vi "DegToDAC (SubVI).vi"(8 "error in (no error)":errorcluster, 10 "R2":dbl format="%#_13g", 11 "Numeric":dbl) -> (0 "error out":errorcluster, 2 "output array":u8[](array[numeric]))   [LabVIEW 2017]
uses:
  <vilib>/express/express arith-compare/Formula/XNode/ExpressFormulaBlockNode.xnode
panel:
  in  "Array":dbl[](array[numeric])=[1202.0, 1288.0, 1472.0, 1472.0, 1379.0]
  out "Result":dbl
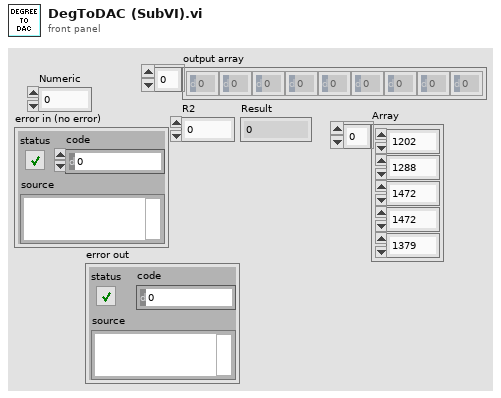
[diagram p1: front panel]
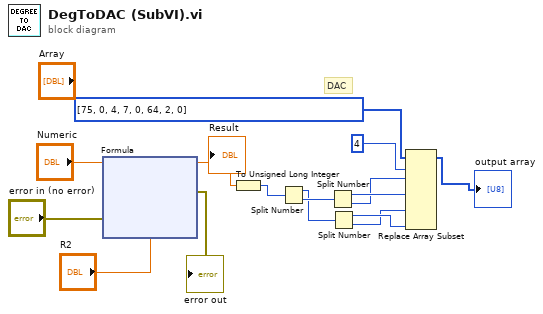
[diagram p0: block diagram]
diagram:
  # "DAC"
  n1 = xnode "Formula"("X2"="R2", "X1"="Numeric", "error in (no error)"="error in (no error)") -> ("Result"=w2:dbl, "error out"=→"error out":errorcluster)
  "Result" <- w2
  n2 = To Unsigned Long Integer(number=w2) -> (unsigned 32bit integer=w3:u32)
  n3 = Split Number(x=w3) -> (hi(x)=w9:u16, lo(x)=w10:u16)
  n4 = Split Number(x=w10) -> (hi(x)=w12:u8, lo(x)=w11:u8)
  n5 = Split Number(x=w9) -> (hi(x)=w14:u8, lo(x)=w13:u8)
  n6 = Replace Array Subset(array=u8[] [75, 0, 4, 7, 0, 64, 2, 0] ("appended array"), new element #1=w11, index #1=4 ("index"), new element #2=w12, new element #3=w13, new element #4=w14) -> (→"output array":u8[])  [unwired: 3 in]
